vi "Desplazamientos_vrl.vi"(6 "Indice":u16, 8 "Rotacion":dbl[](array[numeric])=[1.0, 1.0, 1.0, 1.0], 9 "Translacion":dbl[](array[numeric])=[1.0, 1.0, 1.0], 10 "Escala":dbl[](array[numeric])=[1.0, 1.0, 1.0]) -> (3 "Salida":string[](array[string]))   [LabVIEW 2017]
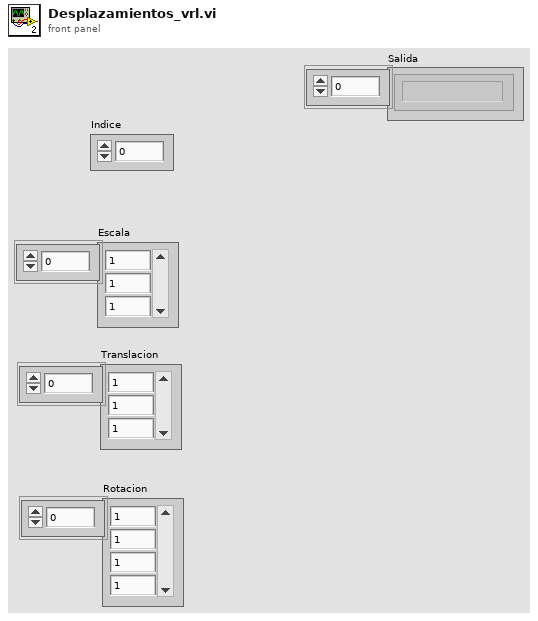
[diagram p1: front panel]
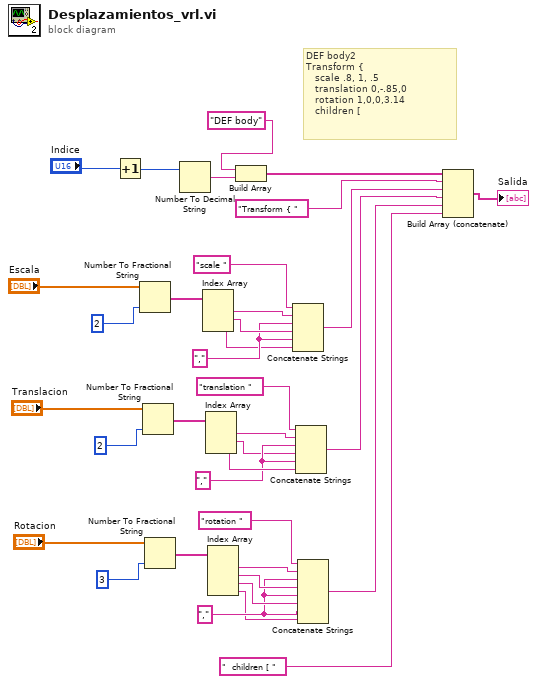
[diagram p0: block diagram]
diagram:
  w6 = ","
  w20 = ","
  w26 = ","
  # "DEF body2\nTransform { \n   scale .8, 1, .5\n   translation 0,-.85,0\n   rotation 1,0,0,3.14\n   children ["
  n1 = Increment(x="Indice") -> (x+1=w35:u16)
  n2 = Number To Fractional String(number="Escala", precision (6)=i16 2) -> (F-format string=w30:string[])  [unwired: 2 in]
  n3 = Number To Fractional String(number="Translacion", precision (6)=i16 2) -> (F-format string=w16:string[])  [unwired: 2 in]
  n4 = Number To Fractional String(number="Rotacion", precision (6)=i16 3) -> (F-format string=w11:string[])  [unwired: 2 in]
  n5 = Number To Decimal String(number=w35) -> (decimal integer string=w34:string)  [unwired: 1 in]
  n6 = Index Array(array=w30) -> (element #1=w28:string, element #2=w27:string, element #3=w25:string)  [unwired: 3 in]
  n7 = Index Array(array=w16) -> (element #1=w18:string, element #2=w19:string, element #3=w21:string)  [unwired: 3 in]
  n8 = Index Array(array=w11) -> (element #1=w9:string, element #2=w8:string, element #3=w7:string, element #4=w5:string)  [unwired: 4 in]
  n9 = Build Array("DEF body", w34) -> (w24:string[])
  n10 = Concatenate Strings("scale ", w28, w26, w27, w26, w25) -> (w22:string)
  n11 = Concatenate Strings("translation ", w18, w20, w19, w20, w21) -> (w4:string)
  n12 = Concatenate Strings("rotation ", w9, w6, w8, w6, w7, w6, w5) -> (w3:string)
  n13 = Build Array (concatenate)(w24, "Transform { ", w22, w4, w3, "  children [ ") -> (→"Salida":string[])
